vi "EXA_acceptCommand_abort.vi"(8 "error in (no error)":errorcluster, 11 "command_abort_Ctl":T1) -> (0 "error out":errorcluster, 2 "function return":i32, 3 "command_abort_Ctl out":T1)   [LabVIEW 2016, in "SALLV_EXA.lvlib"]
doc: "int EXA_shm_acceptCommand_abortLV(EXA_command_abortLV *command_abort_Ctl );"
uses:
  SALLV_EXA.lvlib
  DataTypes/command_abort.ctl
  SALLV_EXA.so
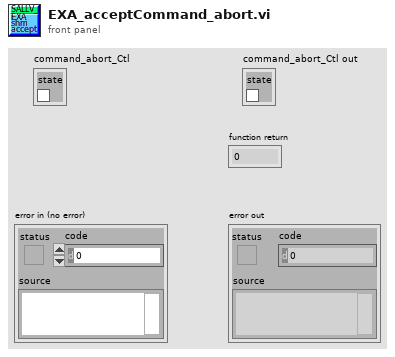
[diagram p1: front panel]
types:
  T1 = typedef "SALLV_EXA.lvlib/command_abort.ctl" = cluster{"state":bool}
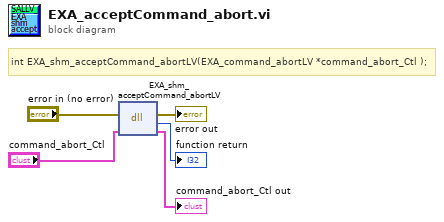
[diagram p0: block diagram]
diagram:
  # "int EXA_shm_acceptCommand_abortLV(EXA_command_abortLV *command_abort_Ctl );"
  n1 = dll-call lib="home/hsundar/TCS/updated_EXA/SALLV_EXA.*" fn="EXA_shm_acceptCommand_abortLV"(error in="error in (no error)", "command_abort_Ctl"="command_abort_Ctl") -> (error out=→"error out":errorcluster, →"function return":i32, "command_abort_Ctl"=→"command_abort_Ctl out":T1)  [unwired: 2 in, 1 out]
